vi "BIN_PAQ_week_num_2_filename.vi"(8 "error in":errorcluster, 9 "num":u64, 10 "ext":string, 11 "TableName":string) -> (0 "error out":errorcluster, 2 "FileName":string)   [LabVIEW 2020, in "Sgraph_lib_V1.lvlib" / "DBAL-BIN.lvclass"]
doc: "Binary PAQ file: numeric file identifier to filename\nThis version constructs the YYYY-WW format"
uses:
  DBAL-BIN.lvclass
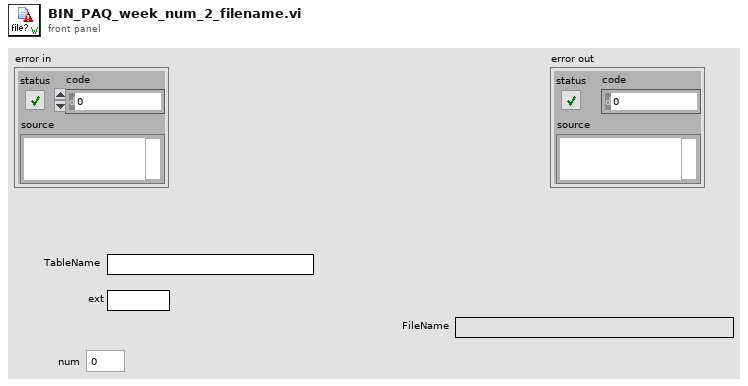
[diagram p1: front panel]
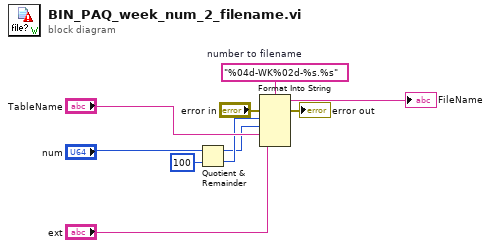
[diagram p0: block diagram]
diagram:
  w9 = "%04d-WK%02d-%s.%s"  # number to filename
  n1 = Quotient & Remainder(x="num", y=u64 100) -> (x-y*floor(x/y)=w1:u64, floor(x/y)=w2:u64)
  n2 = Format Into String(format string=w9, error in="error in", w2, w1, "TableName", "ext") -> (resulting string=→"FileName":string, error out=→"error out":errorcluster)  [unwired: 1 in]
